vi "cmd.vi"() -> ()   [LabVIEW 2019]
uses:
  subVIs/CMD-Ctrl.ctl
  subVIs/Mode-Ctrl.ctl
panel:
  in  "Control Mode 5":T1
  in  "Control Mode 4":T1
  in  "Control Mode 3":T1
  in  "Control Mode 2":T1
  in  "Control Mode":T1
  in  "Reset Commands 10":bool
  in  "Reset Commands 9":bool
  out "?":T2
  out "?":T2
  in  "Reset Commands 8":bool
  in  "Reset Commands 7":bool
  out "?":T2
  out "?":T2
  in  "Reset Commands 6":bool
  in  "Reset Commands 5":bool
  out "?":T2
  out "?":T2
  in  "Reset Commands 4":bool
  in  "Reset Commands 3":bool
  out "?":T2
  out "?":T2
  in  "Reset Commands 2":bool
  in  "Reset Commands":bool
  out "?":T2
  out "?":T2
  # "Main 1"
  # "Main 2"
  # "Fork"
  # "Tube"
  # "UT"
  # "Telescope ShutDown Command"
  # "Alt ShutDown Command"
  # "Az ShutDown Command"
  # "HSB ShutDown Command"
  # "Rotator ShutDown Command"
  # "Adaptor ShutDown Command"
  # "Enclosure ShutDown Command"
  # "MirrorCover ShutDown Command"
  # "Balancin ShutDown Command"
  # "M2 ShutDown Command"
  # "Instrument ShutDown Command"
  # "Control Mode"
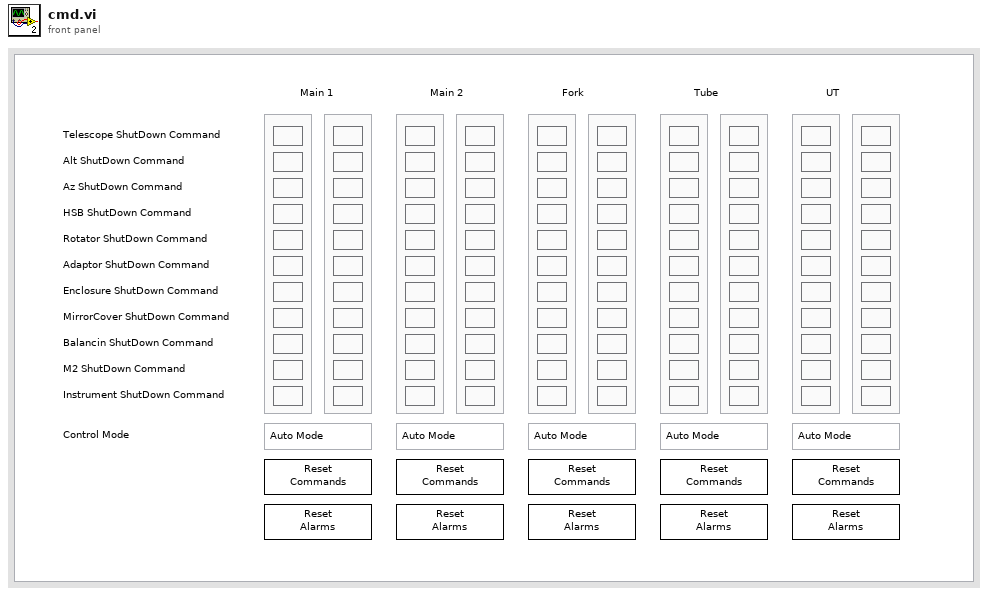
[diagram p1: front panel]
types:
  T1 = typedef "Mode-Ctrl.ctl" = enum16{"Auto Mode", "Maintenance Full Access", "Engineering Mode"}
  T2 = typedef "CMD-Ctrl.ctl" = cluster{"Telescope ShutDown Command":bool, "Alt ShutDown Command":bool, "Az ShutDown Command":bool, "HSB ShutDown Command":bool, "Rotator ShutDown Command":bool, "Adaptor ShutDown Command":bool, "Enclosure ShutDown Command":bool, "MirrorCover ShutDown Command":bool, "Balancing ShutDown Command":bool, "M2 ShutDown Command":bool, "Instrument ShutDown Command":bool}
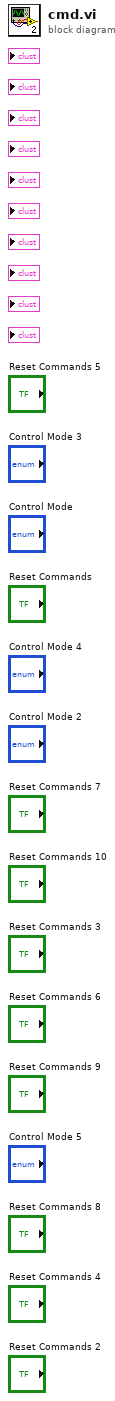
[diagram p0: block diagram]
diagram:
